vi "Slice 3D Cloud.vi"(4 "lower limit (distance)":dbl, 5 "Lower bound (height)":dbl, 6 "upper limit (distance)":dbl, 7 "Upper bound (height)":dbl, 8 "z array in":dbl[](array[numeric]), 9 "y array in":dbl[](array[numeric]), 10 "x array in":dbl[](array[numeric])) -> (2 "Y array":dbl[](array[numeric]), 3 "X array":dbl[](array[numeric]))   [LabVIEW 2010]
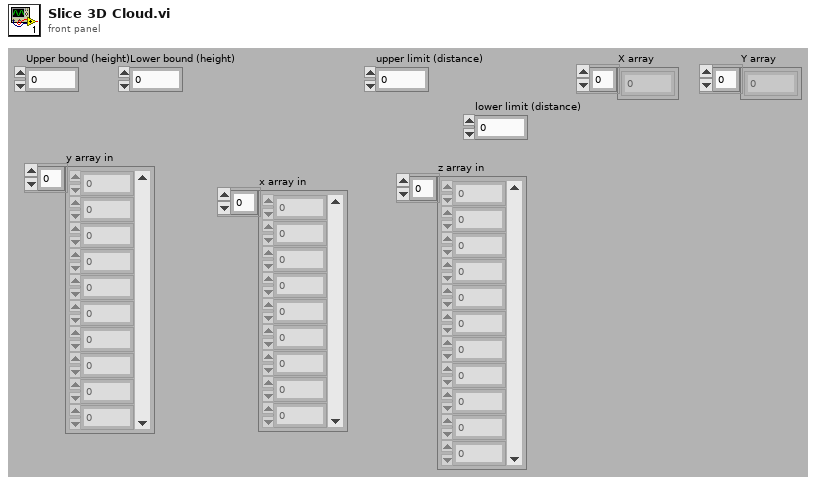
[diagram p1: front panel]
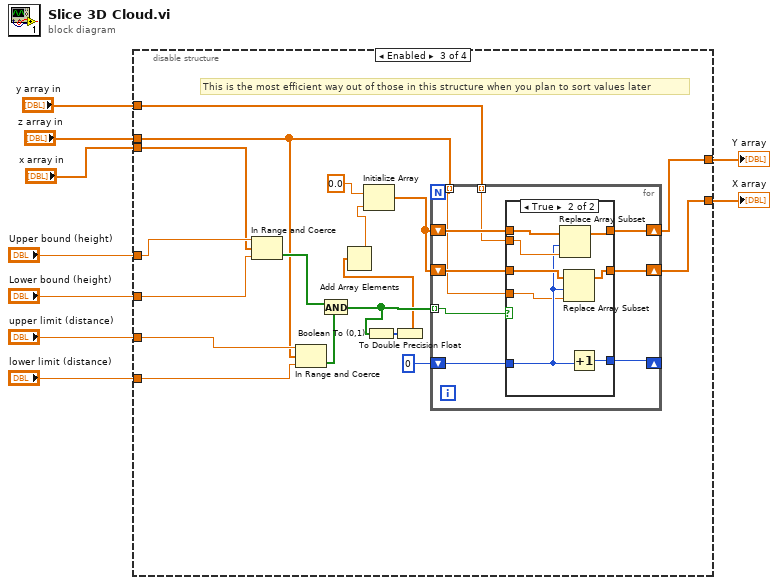
[diagram p0: block diagram]
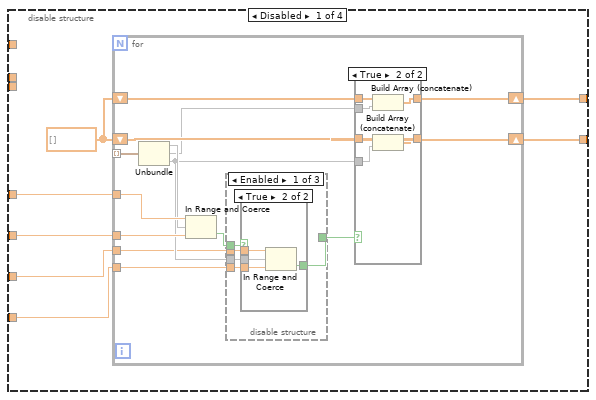
[diagram p2: hidden frame]
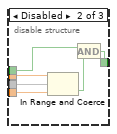
[diagram p4: hidden frame]
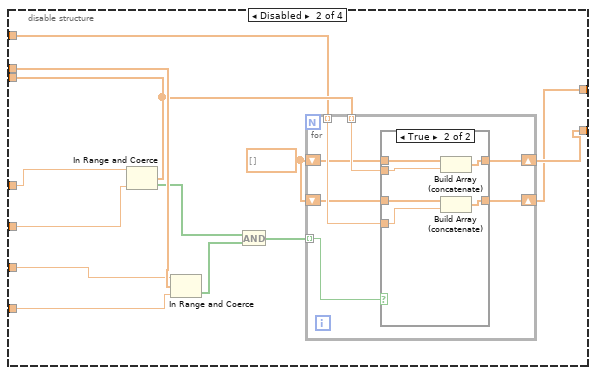
[diagram p7: hidden frame]
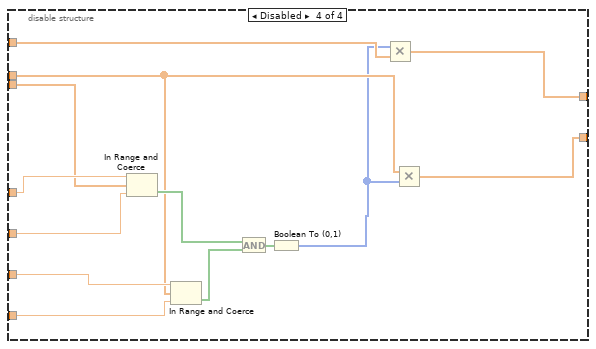
[diagram p10: hidden frame]
diagram:
  n1 = disable-structure shown="Enabled" {
    disable-tunnel: [w16 w57 w87 w127] -> w9
    disable-tunnel: [w15 w58 w86 w123] -> w8
    disable-tunnel: "lower limit (distance)" -> [w14 w64 w98 w131]
    disable-tunnel: "upper limit (distance)" -> [w13 w65 w99 w132]
    disable-tunnel: "Lower bound (height)" -> [w11 w67 w100 w133]
    disable-tunnel: "Upper bound (height)" -> [w10 w68 w101 w134]
    disable-tunnel: "x array in" -> [_ w61 w95 w125]
    disable-tunnel: "z array in" -> [_ w66 w85 w124]
    disable-tunnel: "y array in" -> [_ w60 w94 w126]
    frame Disabled {
      w12 = dbl[] []
      n2 = for {
        tunnel: [w31] -> w17 mode=indexing
        tunnel: w10 -> [w30]
        tunnel: w11 -> [w29]
        shift-right: [w28] -> w16
        shift-left: w12 -> [w27]
        shift-right: [w26] -> w15
        shift-left: w12 -> [w25]
        tunnel: w13 -> [w21]
        tunnel: w14 -> [w20]
        n3 = Unbundle(w31) -> (w24, w23, w22)
        n4 = In Range and Coerce(upper limit=w30, x=w24, lower limit=w29) -> (In Range?=w19:bool)  [unwired: 1 out]
        n5 = disable-structure shown="Enabled" {
          disable-tunnel: w22 -> [w36 w47 _]
          disable-tunnel: w21 -> [w35 w46 _]
          disable-tunnel: w20 -> [w34 w45 _]
          disable-tunnel: w19 -> [w33 w43 _]
          disable-tunnel: [w32 w42 _] -> w18
          frame Enabled {
            n6 = case shown="True" w33 {
              selector: w33 -> [w37 _]
              tunnel: w36 -> [_ w41]
              tunnel: w35 -> [_ w40]
              tunnel: w34 -> [_ w39]
              tunnel: [w37 w38] -> w32
              frame False {
              }
              frame True {
                n7 = In Range and Coerce(upper limit=w40, x=w41, lower limit=w39) -> (In Range?=w38:bool)  [unwired: 1 out]
              }
            }
          }
          frame Disabled {
            n8 = In Range and Coerce(upper limit=w46, x=w47, lower limit=w45) -> (In Range?=w44:bool)  [unwired: 1 out]
            n9 = And(x=w43, y=w44) -> (x .and. y?=w42:bool)
          }
          frame Disabled {
          }
        }
        n10 = case shown="True" w18 {
          tunnel: w23 -> [_ w55]
          tunnel: w22 -> [_ w52]
          tunnel: [w49 w54] -> w28
          tunnel: w27 -> [w49 w53]
          tunnel: [w48 w51] -> w26
          tunnel: w25 -> [w48 w50]
          frame False {
          }
          frame True {
            n11 = Build Array (concatenate)(w53, w55) -> (w54:dbl[])
            n12 = Build Array (concatenate)(w50, w52) -> (w51:dbl[])
          }
        }
      }
    }
    frame Disabled {
      w56 = dbl[] []
      n13 = In Range and Coerce(upper limit=w68, x=w61, lower limit=w67) -> (In Range?=w62:bool[])  [unwired: 1 out]
      n14 = In Range and Coerce(upper limit=w65, x=w66, lower limit=w64) -> (In Range?=w63:bool[])  [unwired: 1 out]
      n15 = And(x=w62, y=w63) -> (x .and. y?=w59:bool[])
      n16 = for {
        tunnel: w61 -> [w75] mode=indexing
        tunnel: w60 -> [w74] mode=indexing
        tunnel: w59 -> [w69] mode=indexing
        shift-right: [w73] -> w58
        shift-left: w56 -> [w71]
        shift-right: [w72] -> w57
        shift-left: w56 -> [w70]
        n17 = case shown="True" w69 {
          tunnel: w75 -> [_ w83]
          tunnel: w74 -> [_ w80]
          tunnel: [w77 w82] -> w73
          tunnel: w71 -> [w77 w81]
          tunnel: [w76 w79] -> w72
          tunnel: w70 -> [w76 w78]
          frame False {
          }
          frame True {
            n18 = Build Array (concatenate)(w81, w83) -> (w82:dbl[])
            n19 = Build Array (concatenate)(w78, w80) -> (w79:dbl[])
          }
        }
      }
    }
    frame Enabled {
      # "This is the most efficient way out of those in this structure when you plan to sort values later"
      n20 = In Range and Coerce(upper limit=w101, x=w95, lower limit=w100) -> (In Range?=w96:bool[])  [unwired: 1 out]
      n21 = In Range and Coerce(upper limit=w99, x=w85, lower limit=w98) -> (In Range?=w97:bool[])  [unwired: 1 out]
      n22 = And(x=w96, y=w97) -> (x .and. y?=w93:bool[])
      n23 = Boolean To (0,1)(Boolean=w93) -> (0, 1=w92:i16[])
      n24 = To Double Precision Float(number=w92) -> (double precision float=w84:dbl[])
      n25 = Add Array Elements(numeric array=w84) -> (sum=w91:dbl)
      n26 = Initialize Array(0.0, w91) -> (w89:dbl[])
      n27 = for {
        tunnel: w85 -> [w103] mode=indexing
        tunnel: w94 -> [w102] mode=indexing
        tunnel: w93 -> [w106] mode=indexing
        shift-right: [w110] -> w87
        shift-left: w89 -> [w108]
        shift-right: [w109] -> w86
        shift-left: w89 -> [w107]
        shift-right: [w104] -> _
        shift-left: 0 -> [w105]
        n28 = case shown="True" w106 {
          tunnel: w102 -> [_ w118]
          tunnel: w103 -> [_ w114]
          tunnel: [w113 w119] -> w110
          tunnel: w108 -> [w113 w120]
          tunnel: [w112 w116] -> w109
          tunnel: w107 -> [w112 w117]
          tunnel: w105 -> [w111 w115]
          tunnel: [w111 w121] -> w104
          frame False {
          }
          frame True {
            n29 = Replace Array Subset(array=w120, new element=w118, index=w115) -> (w119:dbl[])
            n30 = Replace Array Subset(array=w117, new element=w114, index=w115) -> (w116:dbl[])
            n31 = Increment(x=w115) -> (x+1=w121:i32)
          }
        }
      }
    }
    frame Disabled {
      n32 = In Range and Coerce(upper limit=w134, x=w125, lower limit=w133) -> (In Range?=w129:bool[])  [unwired: 1 out]
      n33 = In Range and Coerce(upper limit=w132, x=w124, lower limit=w131) -> (In Range?=w130:bool[])  [unwired: 1 out]
      n34 = And(x=w129, y=w130) -> (x .and. y?=w128:bool[])
      n35 = Boolean To (0,1)(Boolean=w128) -> (0, 1=w122:i16[])
      n36 = Multiply(x=w122, y=w126) -> (x*y=w127:dbl[])
      n37 = Multiply(x=w124, y=w122) -> (x*y=w123:dbl[])
    }
  }
  "Y array" <- w9
  "X array" <- w8
